vi "Find First Valid Removable Drive.vi"() -> (3 "Disk State":T1 {"Used" format="%#.2f"; "Available" format="%#.2f"; "Total" format="%#.2f"})   [LabVIEW 2021]
uses:
  Type Definitions/Disk State.ctl
  Type Definitions/Data Frame.ctl
  Type Definitions/Data Frame Header.ctl
  Type Definitions/Payload Class.ctl
  Type Definitions/Device.ctl
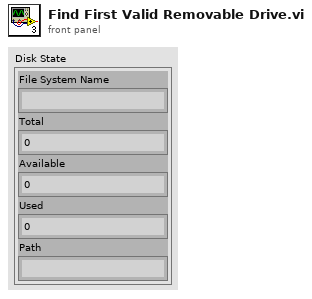
[diagram p1: front panel]
types:
  T1 = typedef "Disk State.ctl" = cluster{"File System Name":string, "Total":sgl, "Available":sgl, "Used":sgl, "Path":string}
  T2 = typedef "Data Frame.ctl" = cluster{"Frame Header":T3, "Payload":string, "CRC":u32}
  T3 = typedef "Data Frame Header.ctl" = cluster{"Sync":u32, "Time":dbl, "Nanosecond Counter":i64, "Payload Class":T4, "Payload ID":u16, "Counter":i32, "Options":u32, "Source":T5, "Destination":T5}
  T4 = typedef "Payload Class.ctl" = enum16{"System State", "Parameters", "Metadata", "Software Monitor", "Data", "Commands"}
  T5 = typedef "Device.ctl" = enum32{"None", "Exec", "Aux1", "Aux2", "Aux3"}
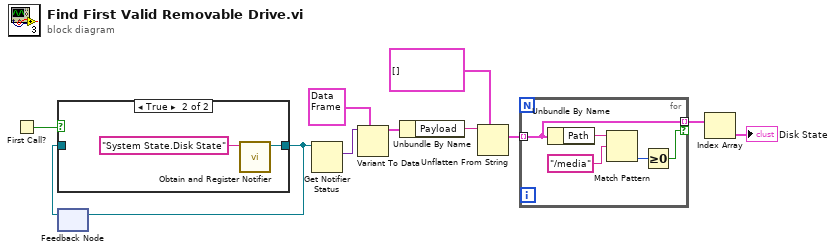
[diagram p0: block diagram]
diagram:
  n1 = First Call?() -> (First Call?: T/F=w9:bool)
  n2 = feedback #1() -> (w10:refnum<notifier>)  [unwired: 1 in]
  n3 = case shown="True" w9 {
    tunnel: [w12 w13] -> w11
    tunnel: w10 -> [w12 _]
    frame False {
    }
    frame True {
      n4 = call "Obtain and Register Notifier.vi"("name (unnamed)"="System State.Disk State") -> ("notifier out"=w13:refnum<notifier>)  [unwired: 8 in, 2 out]
    }
  }
  n5 = feedback-in #1(w11) -> ()
  n6 = Get Notifier Status(notifier=w11) -> (current notification=w2:variant)  [unwired: 1 in, 4 out]
  n7 = Variant To Data(type=T2 {"Frame Header"={"Sync"=0, "Time"=0.0, "Nanosecond Counter"=0, "Payload Class"=enum."System State", "Payload ID"=0, "Counter"=0, "Options"=0, "Source"=enum."None", "Destination"=enum."None"}, "Payload"="", "CRC"=0} ("Frame"), Variant=w2) -> (data=w4:T2)  [unwired: 1 in, 1 out]
  n8 = Unbundle By Name(w4) -> ("Payload"=w5:string)
  n9 = Unflatten From String(type=T1[] [] ("Array"), binary string=w5) -> (value=w1:T1[])  [unwired: 3 in, 2 out]
  n10 = for {
    tunnel: w1 -> [w16] mode=indexing
    tunnel: [w16] -> w7 mode=indexing if=w15
    n11 = Unbundle By Name(w16) -> ("Path"=w19:string)
    n12 = Match Pattern(string=w19, regular expression="/media") -> (offset past match=w17:i32)  [unwired: 1 in, 3 out]
    n13 = Greater Or Equal To 0?(x=w17) -> (x >= 0?=w15:bool)
  }
  n14 = Index Array(array=w7) -> (element=→"Disk State":T1)  [unwired: 1 in]
